vi "SetBasePrices_Washer.vi"(8 "error in":errorcluster, 11 "BasePrices":T1={"SPEED WASH"=0.0, "DELICATES"=0.0, "WHITES"=9.75, "COLORS"=0.0, "TOWELS"=0.0, "SANITIZE"=0.0} {"SPEED WASH" min=0.0 max=9.75 step=0.25; "DELICATES" min=0.0 max=9.75 step=0.25; "WHITES" min=0.0 max=9.75 step=0.25; "COLORS" min=0.0 max=9.75 step=0.25; "TOWELS" min=0.0 max=9.75 step=0.25; "SANITIZE" min=0.0 max=9.75 step=0.25}) -> (0 "error out":errorcluster, 3 "PriceData":string)   [LabVIEW 2021]
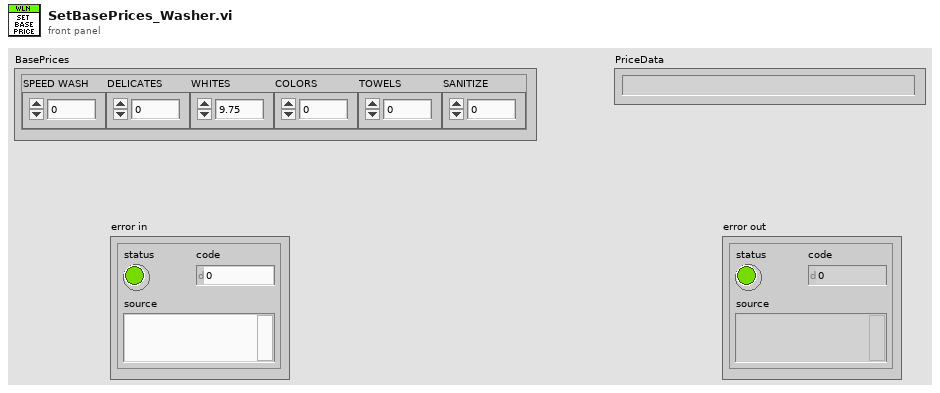
[diagram p1: front panel]
types:
  T1 = cluster{"SPEED WASH":dbl, "DELICATES":dbl, "WHITES":dbl, "COLORS":dbl, "TOWELS":dbl, "SANITIZE":dbl}
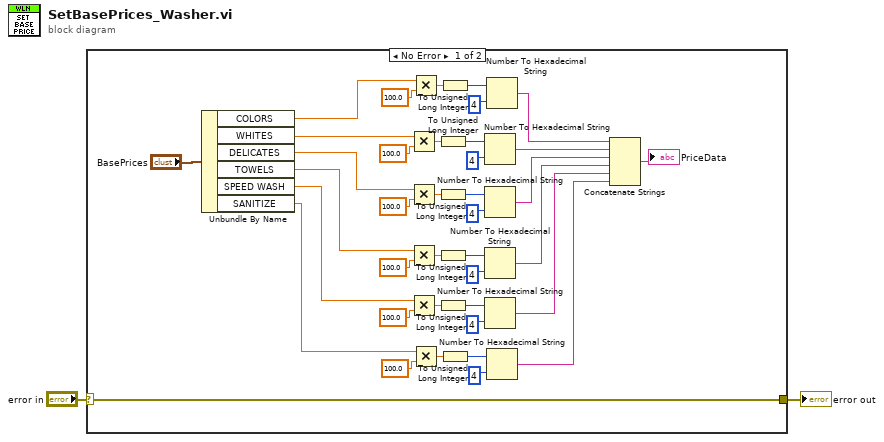
[diagram p0: block diagram]
diagram:
  n1 = case shown="No Error" "error in" {
    selector: "error in" -> [w16 w42]
    tunnel: [w16 w42] -> w1
    frame No Error {
      n2 = Unbundle By Name("BasePrices") -> ("COLORS"=w20:dbl, "WHITES"=w19:dbl, "DELICATES"=w18:dbl, "TOWELS"=w17:dbl, "SPEED WASH"=w4:dbl, "SANITIZE"=w3:dbl)
      n3 = Multiply(x=w19, y=100.0) -> (x*y=w36:dbl)
      n4 = Multiply(x=w18, y=100.0) -> (x*y=w31:dbl)
      n5 = Multiply(x=w17, y=100.0) -> (x*y=w28:dbl)
      n6 = Multiply(x=w4, y=100.0) -> (x*y=w12:dbl)
      n7 = Multiply(x=w20, y=100.0) -> (x*y=w39:dbl)
      n8 = Multiply(x=w3, y=100.0) -> (x*y=w9:dbl)
      n9 = To Unsigned Long Integer(number=w36) -> (unsigned 32bit integer=w37:u32)
      n10 = To Unsigned Long Integer(number=w31) -> (unsigned 32bit integer=w30:u32)
      n11 = To Unsigned Long Integer(number=w28) -> (unsigned 32bit integer=w29:u32)
      n12 = To Unsigned Long Integer(number=w12) -> (unsigned 32bit integer=w11:u32)
      n13 = To Unsigned Long Integer(number=w39) -> (unsigned 32bit integer=w38:u32)
      n14 = To Unsigned Long Integer(number=w9) -> (unsigned 32bit integer=w10:u32)
      n15 = Number To Hexadecimal String(1:i16 4 ("width (-)"), 2:w37) -> (0:w24:string)
      n16 = Number To Hexadecimal String(1:i16 4 ("width (-)"), 2:w30) -> (0:w23:string)
      n17 = Number To Hexadecimal String(1:i16 4 ("width (-)"), 2:w29) -> (0:w22:string)
      n18 = Number To Hexadecimal String(1:i16 4 ("width (-)"), 2:w11) -> (0:w6:string)
      n19 = Number To Hexadecimal String(1:i16 4 ("width (-)"), 2:w38) -> (0:w25:string)
      n20 = Number To Hexadecimal String(1:i16 4 ("width (-)"), 2:w10) -> (0:w5:string)
      n21 = Concatenate Strings(w25, w24, w23, w22, w6, w5) -> (→"PriceData":string)
    }
    frame Error {
    }
  }
  "error out" <- w1
